vi "Project.vi"() -> ()   [LabVIEW 2014]
uses:
  Cntrls/Scada Mode.ctl
  Cntrls/Process Variable.ctl
  Cntrls/Manipulated Variable.ctl
  Cntrls/Message Cluster.ctl
  <vilib>/Utility/file.llb/Write To Spreadsheet File (DBL).vi
panel:
  in  "Начать запись":bool
  out "Waveform Graph 2":dbl[](graph)
  out "real-time, msec":dbl format="%#_4g"
  out "Initial graph and object identification graph":cluster{"all rows":dbl[], "all rows":dbl[]}[](graph) caption="Исходный\n график и\n график\n идентификации объекта"
  in  "dt, msec":u32=200
  in  "SCADA Start":bool
  in  "Exit Button":bool
  out "State":string caption="Display"
  in  "Tab Control":enum32{"SCADA", "Autotuning Controller"}(tab)
  in  "Pump MV":dbl(slide) scale=0.0..1.0
  in  "SCADA Configuration":T4={"HMI Selection"=enum."None", "Control Loop Mode"=enum."None", "Process Variable (PV)"=enum."Level", "Manipulated Variable (MV)"=enum."Pump"}
  out "PV, Level, [cm]":dbl
  in  "SP, Level Control, [cm]":dbl min=0.0 max=100.0 step=0.1
  in  "SP, Flow Control 2, [l/m]":dbl min=0.0 max=100.0 step=0.1
  out "PV, Flow meter 2, [l/m]":dbl format="%#_2g"
  in  "SP, Flow Control 1, [l/m]":dbl min=0.0 max=100.0 step=0.1
  in  "Valve 1 MV":dbl min=0.0 max=1.0 step=0.01
  out "Valve 1 Mode":enum16{"Auto", "Man", "Error"}(ring)
  out "Valve 2 Mode":enum16{"Auto", "Man", "Error"}(ring)
  in  "Working on closed valve 1 On/Off":bool
  out "LLA":bool
  in  "HHAS On/Off":bool
  out "HHA":bool
  in  "LLAS On/Off":bool
  in  "Valve 2 MV":dbl min=0.0 max=1.0 step=0.01
  out "OP, Valve 2%":dbl caption="%"
  out "?":string
  out "?":string
  out "Slide":dbl(slide) scale=0.0..30.0
  out "OP, Valve 1 %":dbl
  out "OP, Pump":dbl
  out "PV, Flow meter 1, [l/m]":dbl
  out "Pump Mode":enum16{"Auto", "Man", "Error"}(ring)
  out "Level N":dbl
  out "Flow meter N1":dbl
  out "Flow meterN2":dbl
  in  "Set PID Coeffs To PLC":bool
  in  "Start Identification":bool
  in  "Start Autotune":bool
  in  "Start Acquisition":bool
  in  "Control action level":dbl
  in  "Identified First - Order process + Deadtime transfer function":T5
  in  "P1":dbl
  in  "P2":dbl
  in  "P3":dbl
  in  "Transient response \nrecord ends in repetitions":dbl=50.0 min=50.0 max=300.0 step=1.0 format="%#_13g"
  in  "Select Identification Method":enum16{"Transient Response", "Proni"}(ring)
  in  "IMC filter value\n(PI > 0,7; PID > 1,7)":dbl(slide) step=0.1 scale=0.7..10.0
  in  "Select Autotune Method":enum32{"Ziegler  -  Nichols", "IMC", "Amigo"}(ring)
  in  "Type of controller":enum16{"PID", "PI", "P"}(ring)
  in  "Prony approximation zone":enum16{"3/4 zone", "1/2 zone", "1/3 zone"}(ring)
  out "Аverage error":dbl
  out "Transient response database":dbl[][](array[numeric])
  out "Identification X":dbl[](array[numeric])
  in  "Process Variable (PV)":T2
  in  "Manipulated Variable (MV)":T3
  out "Waveform Graph":dbl[](graph)
  # "Valve 2"
  # "Valve 2"
  # "Mode"
  # "[%]"
  # "Valve 1"
  # "MV"
  # "Mode"
  # "[%]"
  # "MV"
  # "PUMP"
  # "Mode"
  # "MV"
  # "Config Control Loop"
  # "Transient response database record & Transfer function identification configuration"
  # "Identification Configuration"
  # "Select variables"
  # "Record parameters"
  # "PID Autotune configuration & Controller parametrs"
  # "Controller parameters"
  # "Autotune selection"
  # "Created by ATM-21-01 (Dem, Shish, Destructor)"
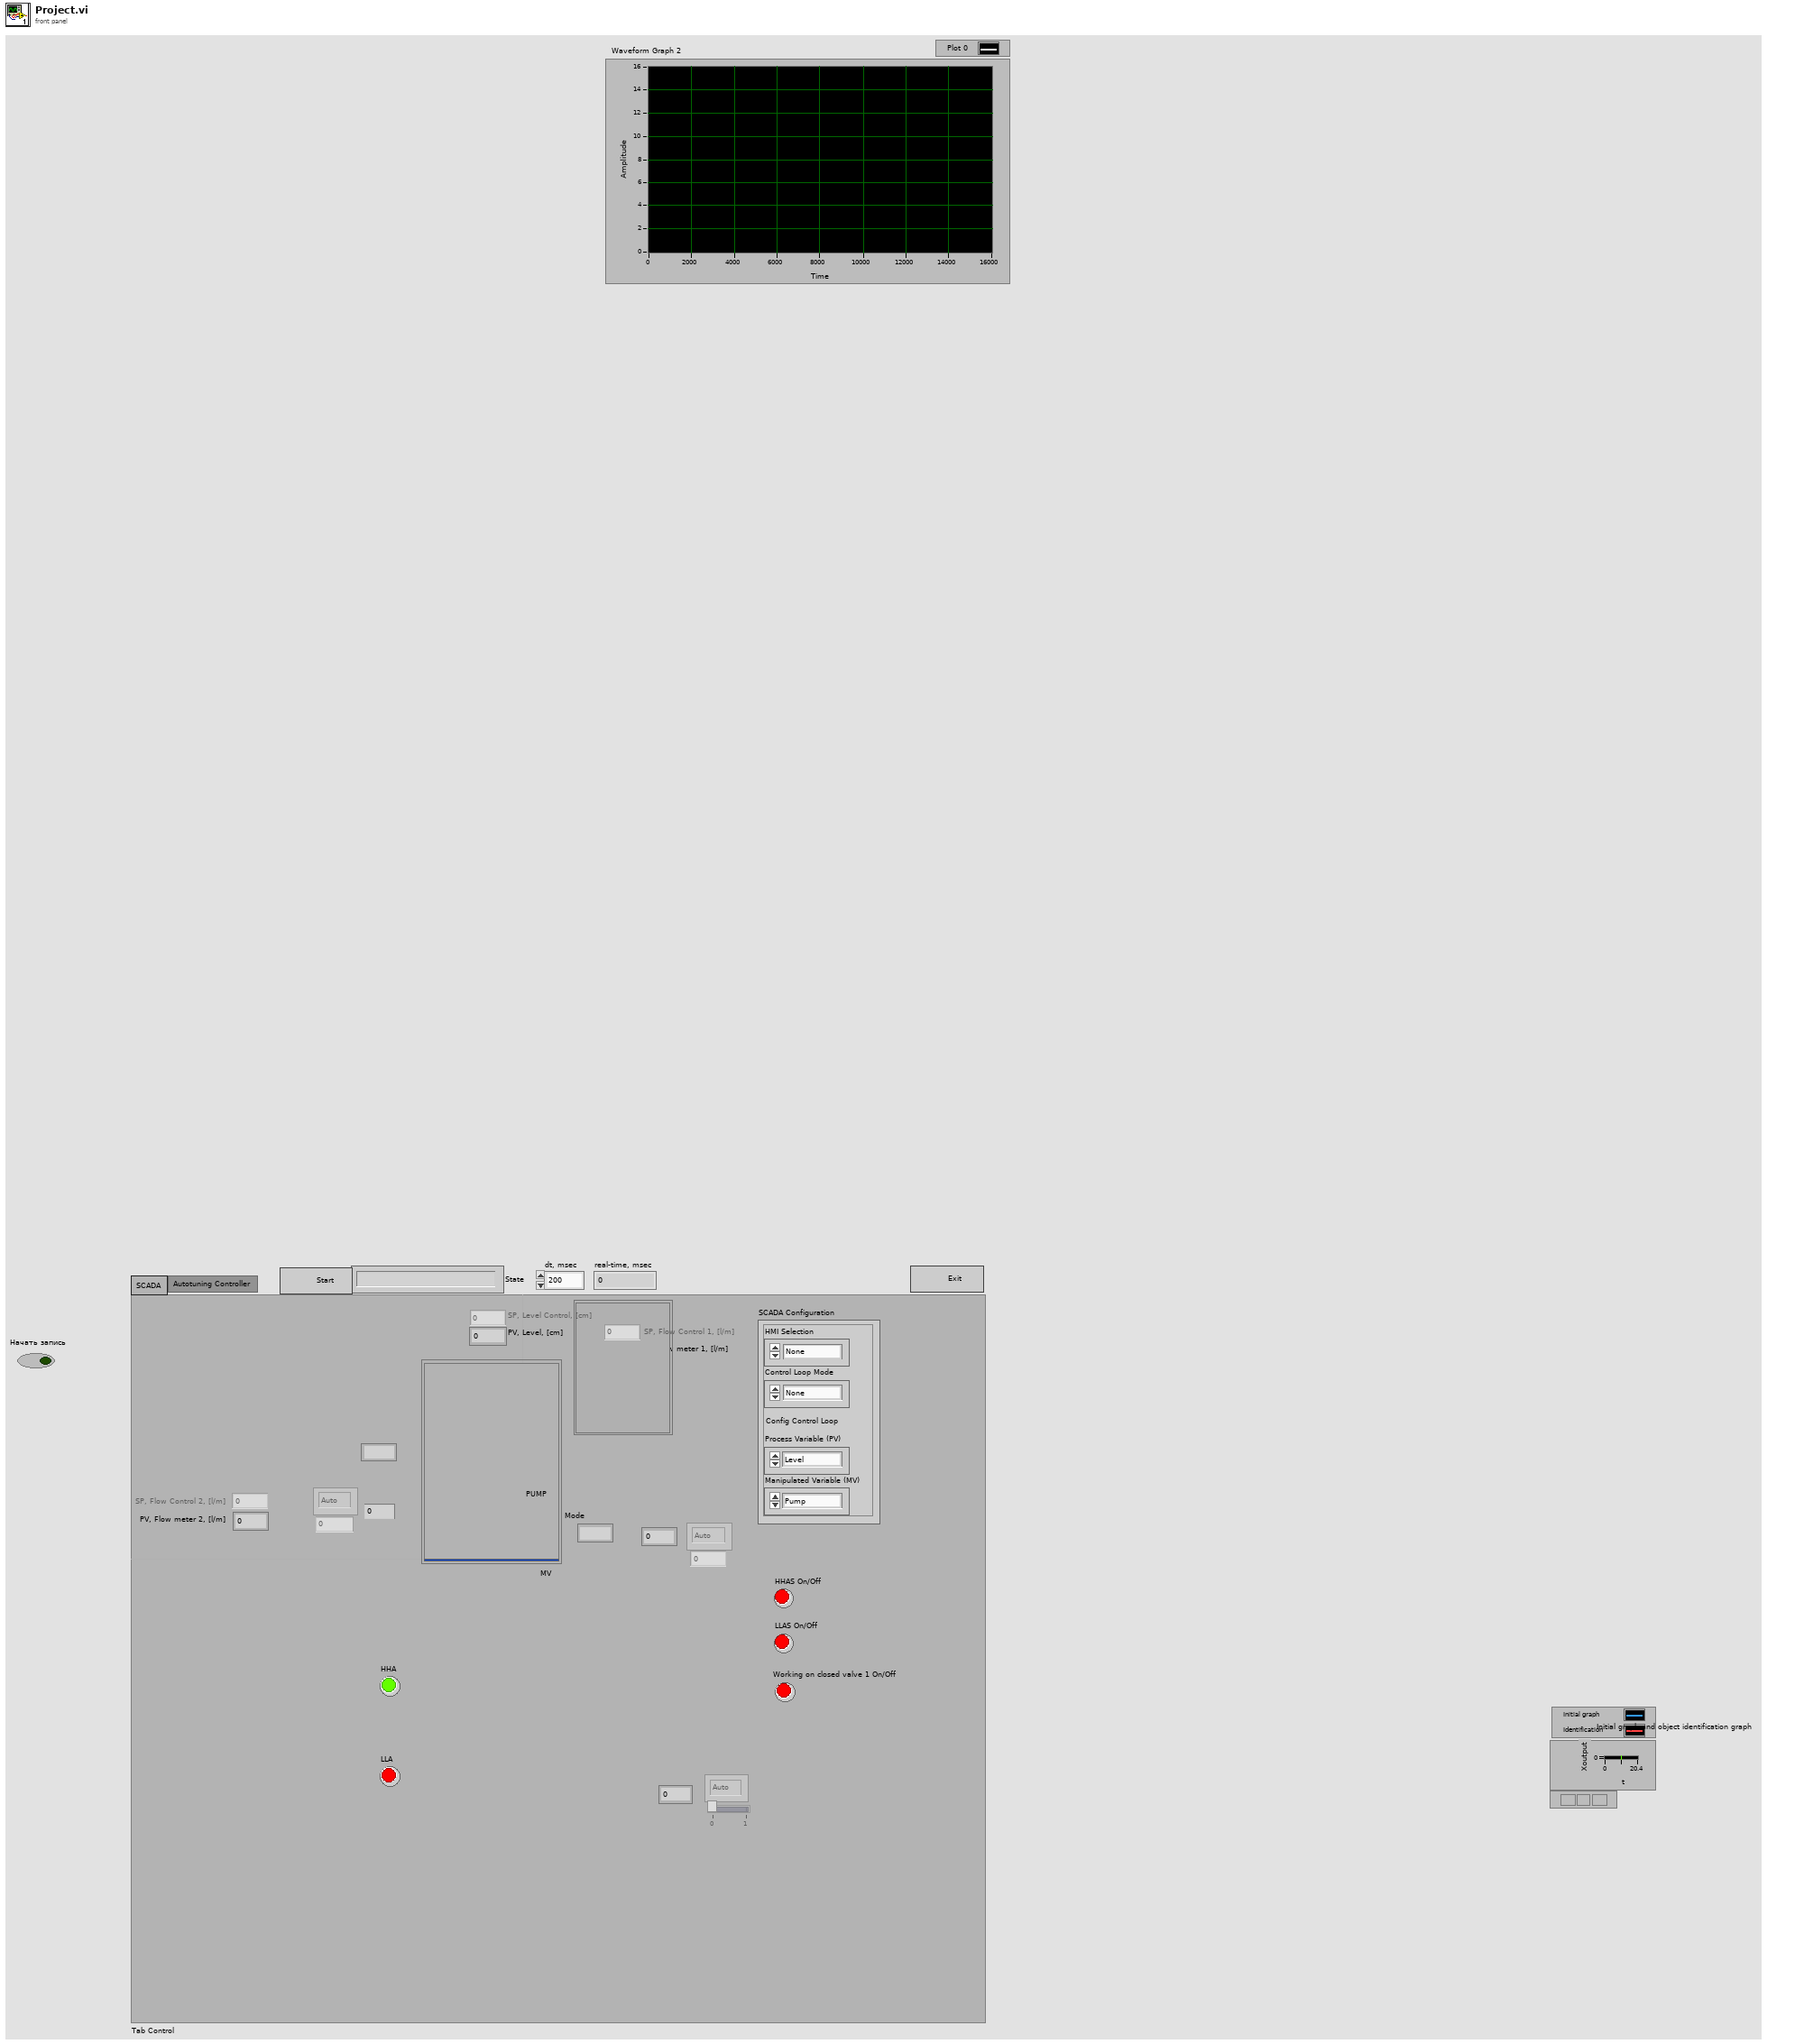
[diagram p1: front panel]
types:
  T1 = typedef "Scada Mode.ctl" = enum16{"None", "Manual", "Auto"}
  T2 = typedef "Process Variable.ctl" = enum16{"None", "Level", "Flow 1", "Flow 2"}
  T3 = typedef "Manipulated Variable.ctl" = enum16{"None", "Pump", "Valve 1", "Valve 2"}
  T4 = cluster{"HMI Selection":enum16{"Panel", "Scada", "Remote Control", "None"}, "Control Loop Mode":T1, "Process Variable (PV)":T2, "Manipulated Variable (MV)":T3}
  T5 = cluster{"K - gain coefficient":dbl, "tau - delay time":dbl, "T - time constant":dbl}
  T6 = typedef "Message Cluster.ctl" = cluster{"Enum":variant, "Message":string}
  T7 = enum16{"Read", "Write", "ReadWrite", "BufferedRead", "BufferedReadWrite"}
  T8 = cluster{"PVs":refnum<k13>[], "OPs":refnum<k13>[], "SPs":refnum<k13>[], "MVs":refnum<k13>[], "Controls":refnum<k13>[], "Indicators":refnum<k13>[], "Protection":refnum<k13>[], "PVs Norm ":refnum<k13>[]}
  T9 = enum16{"Panel", "Scada", "Remote Control", "None"}
  T10 = enum8{"Enabled", "Disabled", "Disabled and Grayed Out"}
  T11 = cluster{"к - gain coefficient":dbl, "tau -delay time":dbl, "T - time constant":dbl}
  T12 = cluster{"Data For Ident From OPC":dbl[], "Data For Ident From OPC":dbl[]}[]
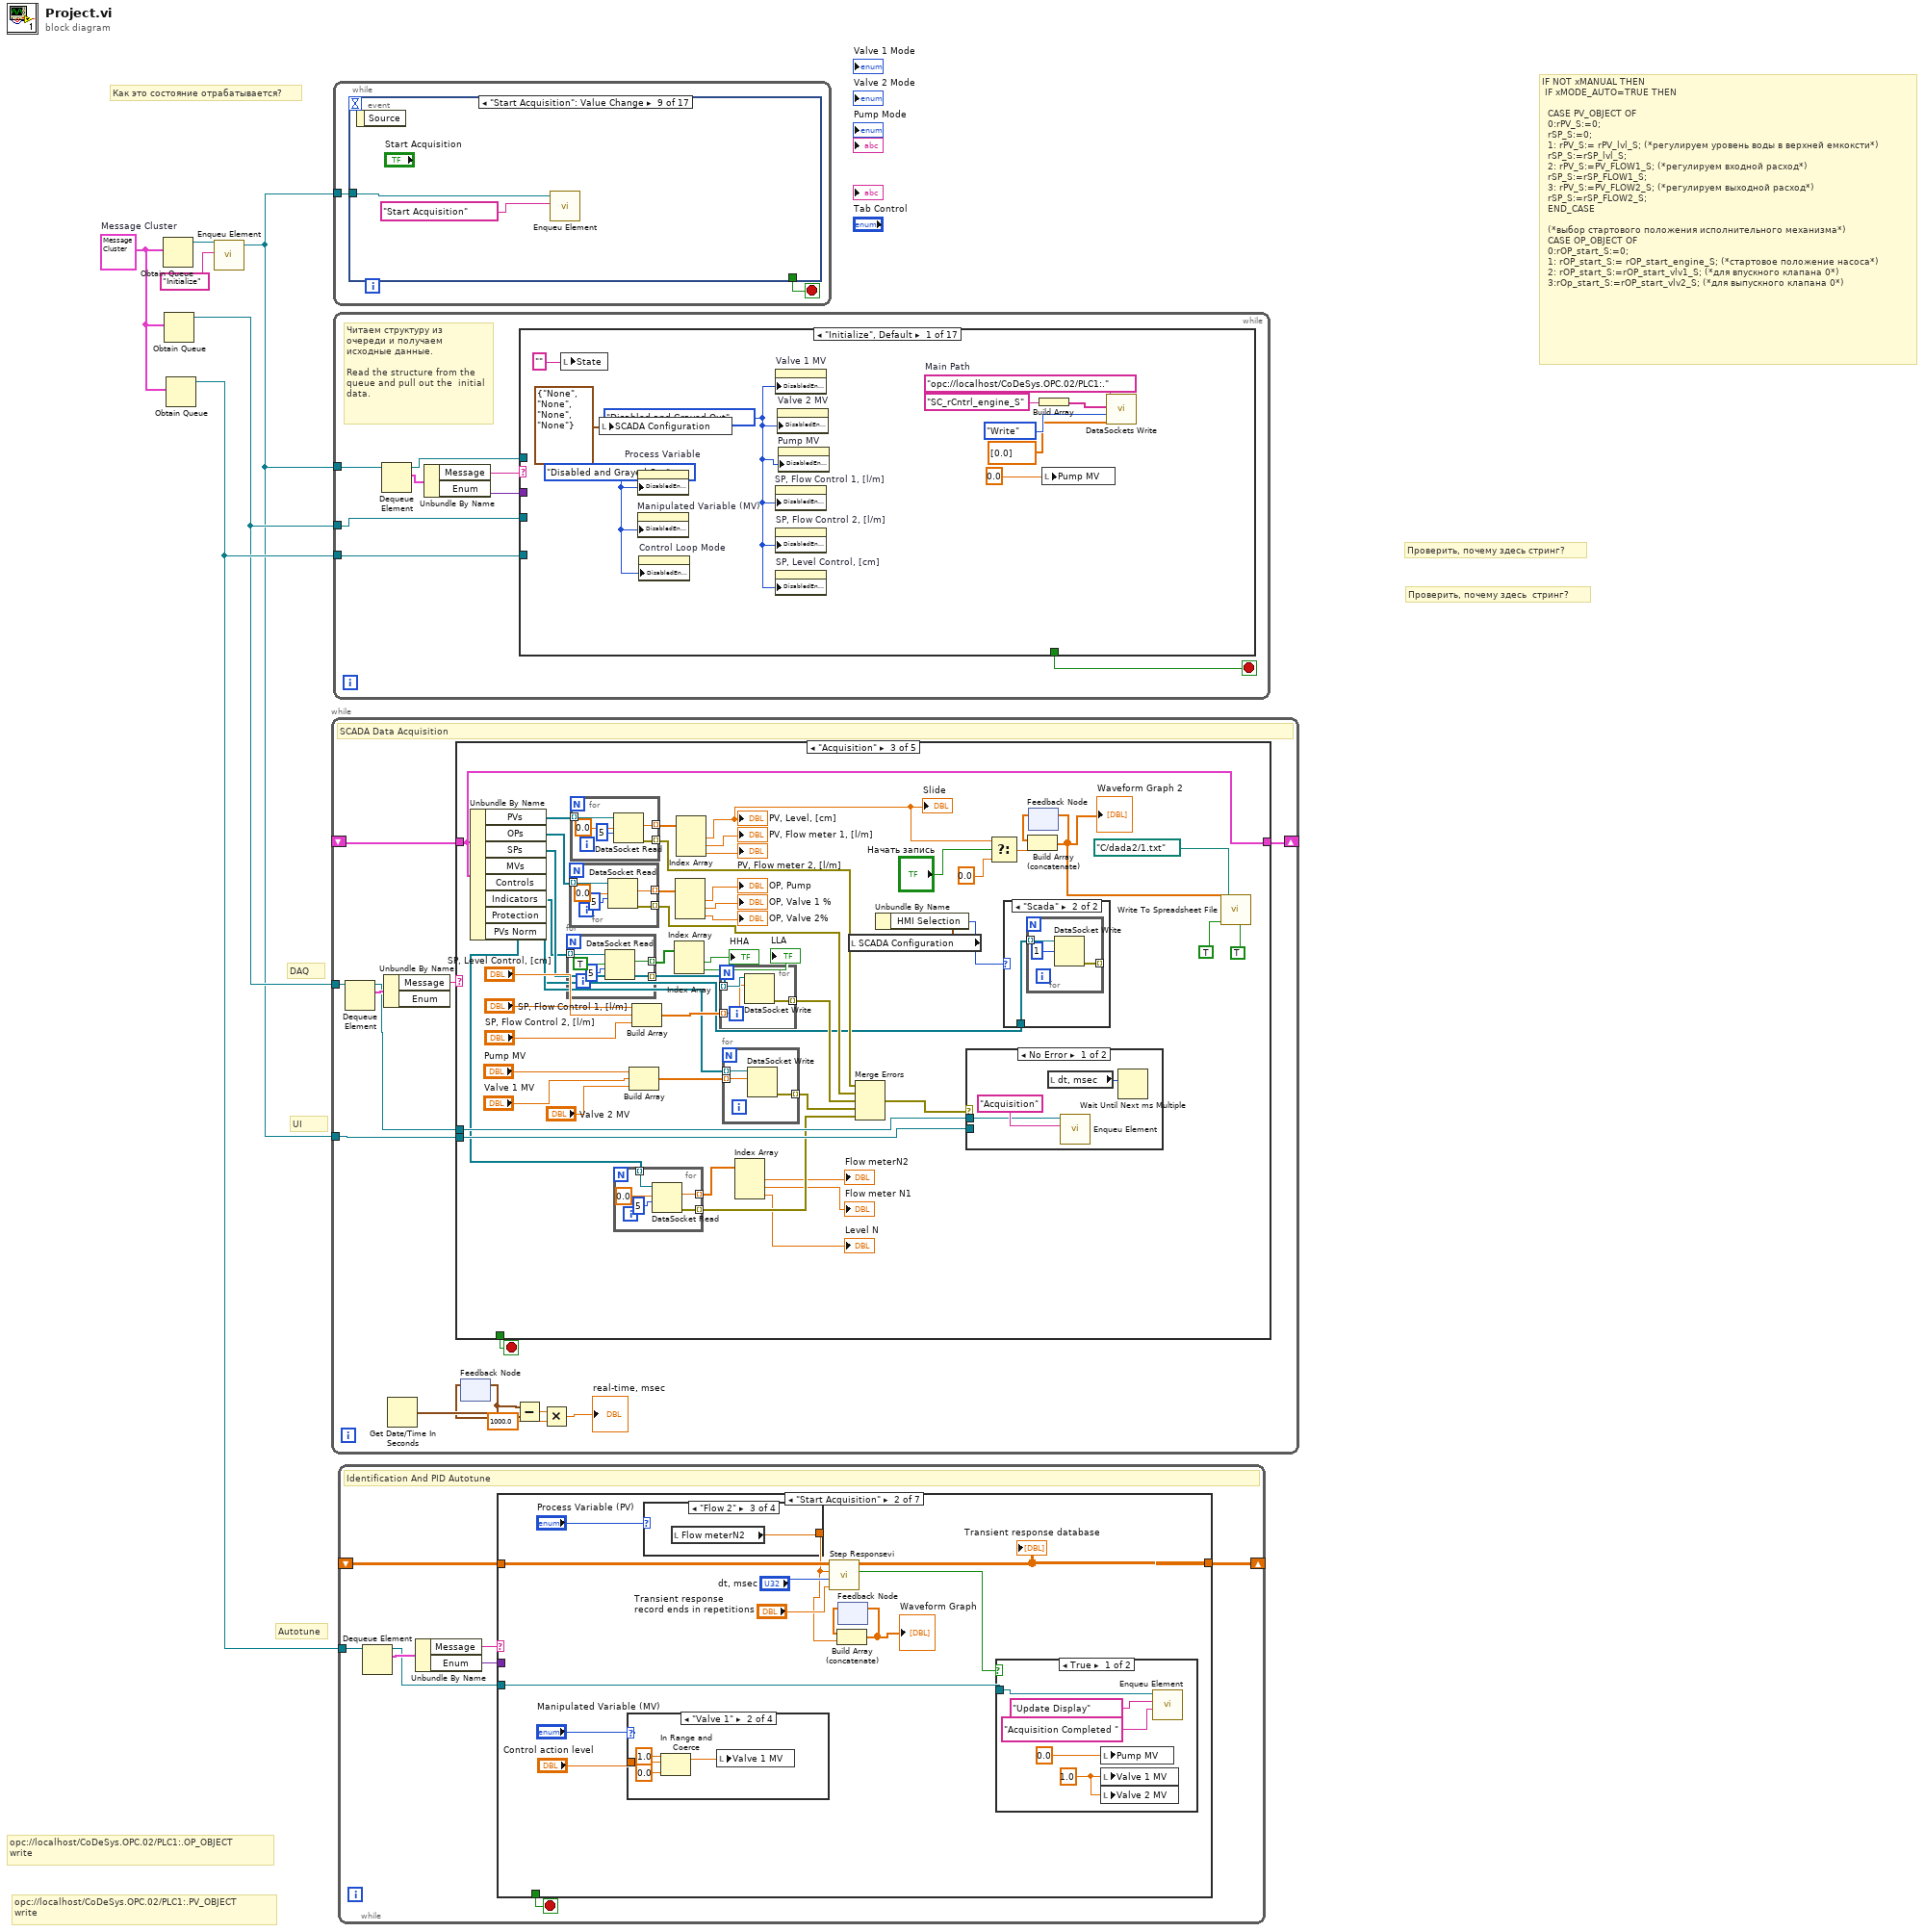
[diagram p0: block diagram]
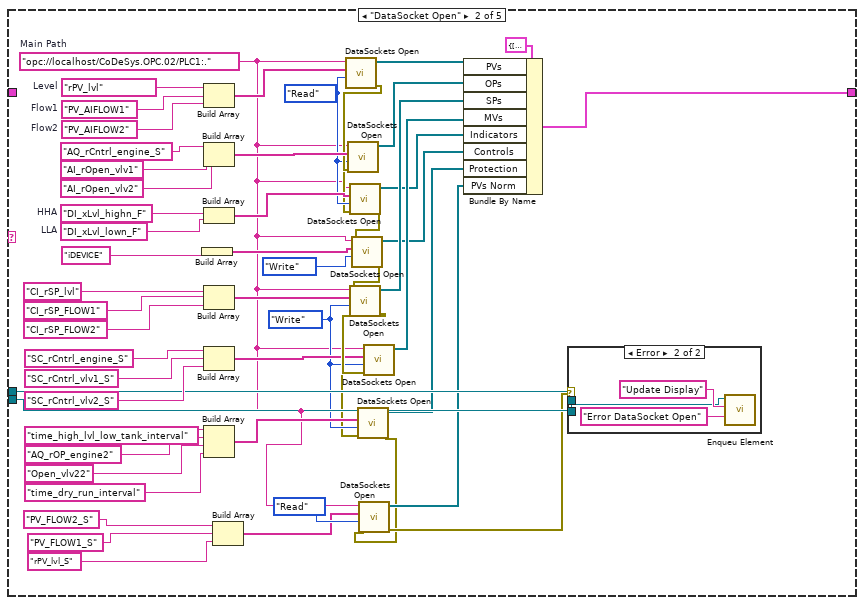
[diagram p3: hidden frame]
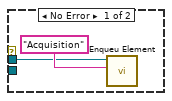
[diagram p4: hidden frame]
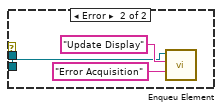
[diagram p6: hidden frame]
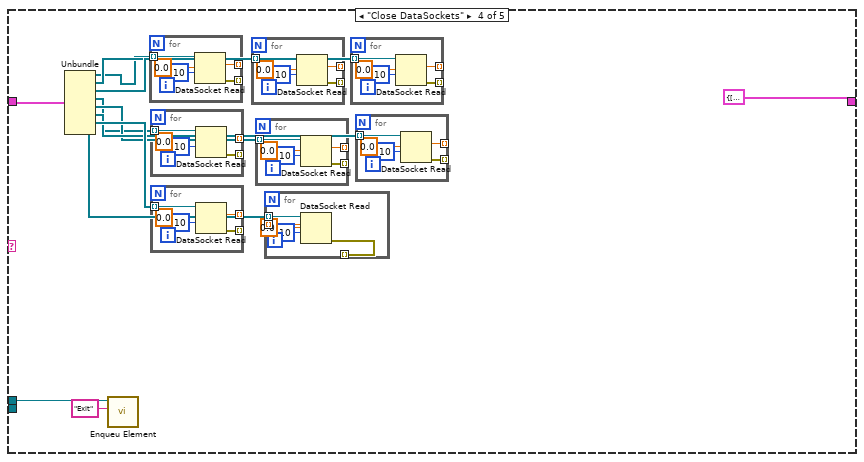
[diagram p7: hidden frame]
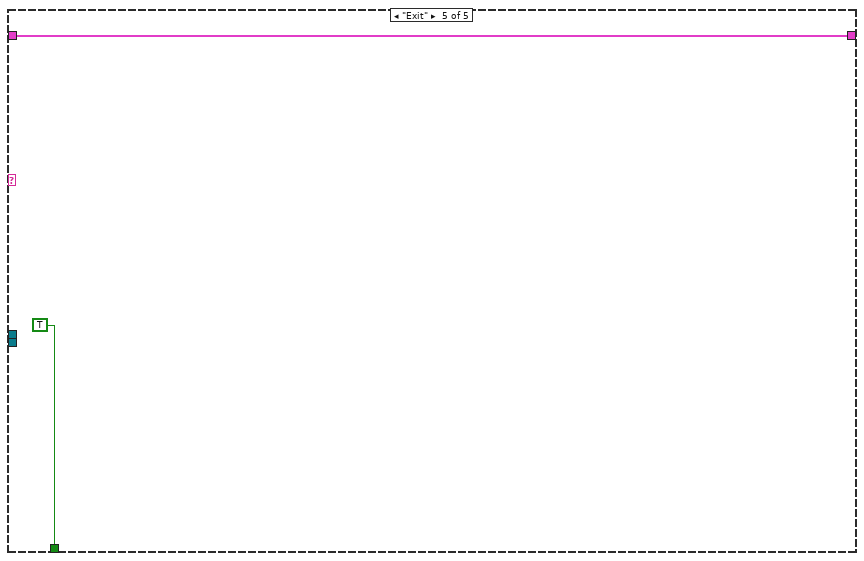
[diagram p8: hidden frame]
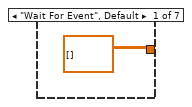
[diagram p9: hidden frame]
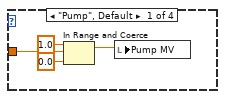
[diagram p10: hidden frame]
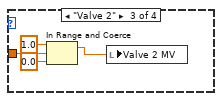
[diagram p11: hidden frame]
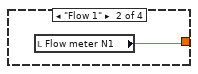
[diagram p14: hidden frame]
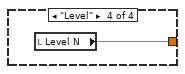
[diagram p15: hidden frame]
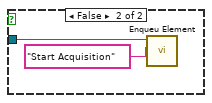
[diagram p16: hidden frame]
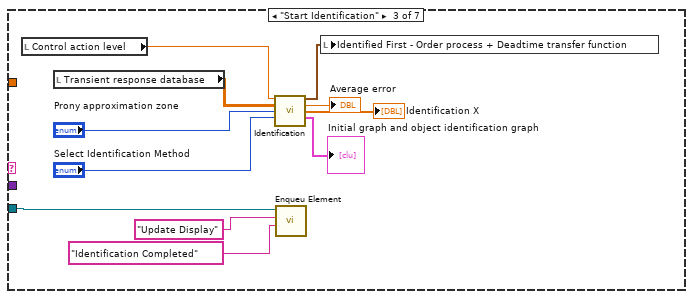
[diagram p17: hidden frame]
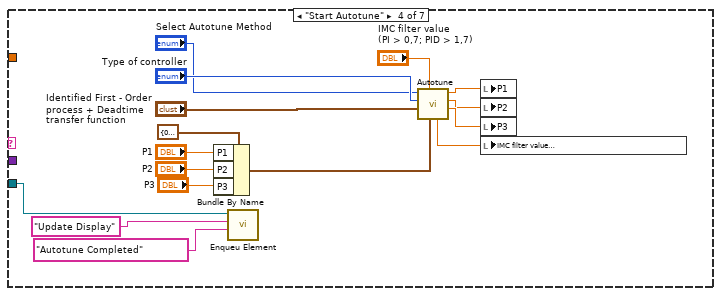
[diagram p18: hidden frame]
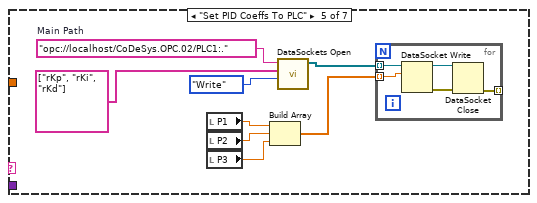
[diagram p19: hidden frame]
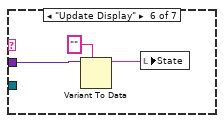
[diagram p20: hidden frame]
diagram:
  w3 = T6 {"Enum"=variant, "Message"=""}  # Message Cluster
  # "Проверить, почему здесь  стринг?"
  # "Проверить, почему здесь стринг?"
  # "IF NOT xMANUAL THEN\n\tIF xMODE_AUTO=TRUE THEN\n\n\t\tCASE PV_OBJECT OF\n\t\t0:rPV_S:=0;\n\t\trSP_S:=0;\n\t\t1: rPV_S:= rPV_lvl_S; (*регулируем уровень воды в верхней емкоксти*)\n\t\trSP_S:=rSP_lvl_S;\n\t\t2: rPV_S:=PV_FLOW1_S; (*регулируем входной расход*)\n\t\trSP_S:=rSP_FLOW1_S;\n\t\t3: rPV_S:=PV_FLOW2_S; (*регулируем выходной расход*)\n\t\trSP_S:=rSP_FLOW2_S;\n\t\tEND_CASE\n\n\t\t(*выбор стартового положения исполнительного механизма*)\n\t\tCASE OP_OBJECT OF\n\t\t0:rOP_start_S:=0;\n\t\t1: rOP_start_S:= rOP_start_engine_S; (*стартовое положение насоса*)\n\t\t2: rOP_start_S:=rOP_start_vlv1_S; (*для впускного клапана 0*)\n\t\t3:rOp_start_S:=rOP_start_vlv2_S; (*для выпускного клапана 0*)"
  # "Autotune"
  # "DAQ"
  # "UI"
  # "opc://localhost/CoDeSys.OPC.02/PLC1:.PV_OBJECT\nwrite"
  # "opc://localhost/CoDeSys.OPC.02/PLC1:.OP_OBJECT\nwrite"
  # "Как это состояние отрабатывается?"
  n1 = Obtain Queue(element data type=w3) -> (queue out=w5:refnum<queue>)  [unwired: 4 in, 2 out]
  n2 = Obtain Queue(element data type=w3) -> (queue out=w2:refnum<queue>)  [unwired: 4 in, 2 out]
  n3 = Obtain Queue(element data type=w3) -> (queue out=w6:refnum<queue>)  [unwired: 4 in, 2 out]
  n4 = call "Enqueu Element.vi"("Message"="Initialize", "Queue in"=w5) -> ("queue out"=w1:refnum<queue>)  [unwired: 9 in]
  n5 = while {
    tunnel: w2 -> [w17]
    shift-right: [w16] -> _
    shift-left: _ -> [w15]
    tunnel: w1 -> [w13]
    stop <- w14 stop-if-true
    # "SCADA Data Acquisition"
    n6 = Dequeue Element(queue=w17) -> (queue out=w12:refnum<queue>, element=w19:T6)  [unwired: 2 in, 2 out]
    n7 = Unbundle By Name(w19) -> ("Message"=w18:string)  [unwired: 1 out]
    n8 = Get Date/Time In Seconds() -> (seconds since 1Jan1904=w11:timestamp)
    n9 = case shown="\"Acquisition\"" w18 {
      tunnel: [w20 w66 w129 T8 {"PVs"=[], "OPs"=[], "SPs"=[], "MVs"=[], "Controls"=[], "Indicators"=[], "Protection"=[], "PVs Norm "=[]} ("cluster") w218] -> w16
      tunnel: w12 -> [_ w65 w105 w167 _]
      tunnel: w15 -> [w20 _ w129 w169 w218]
      tunnel: [_ _ _ _ TRUE] -> w14
      tunnel: w13 -> [_ w58 w104 _ _]
      frame "Wait For Event", Default {
      }
      frame "DataSocket Open" {
        w45 = "DI_xLvl_lown_F"  # LLA
        w46 = "DI_xLvl_highn_F"  # HHA
        w35 = T7."Write" ("mode")
        w42 = T7."Read" ("mode")
        w23 = "opc://localhost/CoDeSys.OPC.02/PLC1:."  # Main Path
        w56 = "PV_AIFLOW2"  # Flow2
        w57 = "PV_AIFLOW1"  # Flow1
        w75 = "rPV_lvl"  # Level
        n10 = Build Array("iDEVICE") -> (w51:string[])
        n11 = Build Array(w75, w57, w56) -> (w74:string[])
        n12 = Build Array("AQ_rCntrl_engine_S", "AI_rOpen_vlv1", "AI_rOpen_vlv2") -> (w63:string[])
        n13 = Build Array(w46, w45) -> (w43:string[])
        n14 = Build Array("CI_rSP_lvl", "CI_rSP_FLOW1", "CI_rSP_FLOW2") -> (w55:string[])
        n15 = Build Array("SC_rCntrl_engine_S", "SC_rCntrl_vlv1_S", "SC_rCntrl_vlv2_S") -> (w53:string[])
        n16 = Build Array("time_high_lvl_low_tank_interval", "AQ_rOP_engine2", "Open_vlv22", "time_dry_run_interval") -> (w36:string[])
        n17 = Build Array("PV_FLOW2_S", "PV_FLOW1_S", "rPV_lvl_S") -> (w24:string[])
        n18 = call "DataSockets Open.vi"("mode"=w42, "Variables"=w74, "Main Path"=w23) -> ("error out"=w62:errorcluster, "Array"=w64:refnum<k13>[])  [unwired: 7 in]
        n19 = call "DataSockets Open.vi"("error IO"=w62, "mode"=w42, "Variables"=w63, "Main Path"=w23) -> ("error out"=w41:errorcluster, "Array"=w61:refnum<k13>[])  [unwired: 6 in]
        n20 = call "DataSockets Open.vi"("error IO"=w41, "mode"=w42, "Variables"=w43, "Main Path"=w23) -> ("error out"=w31:errorcluster, "Array"=w40:refnum<k13>[])  [unwired: 6 in]
        n21 = call "DataSockets Open.vi"("error IO"=w31, "mode"=T7."Write", "Variables"=w51, "Main Path"=w23) -> ("error out"=w30:errorcluster, "Array"=w44:refnum<k13>[])  [unwired: 6 in]
        n22 = call "DataSockets Open.vi"("error IO"=w30, "mode"=w35, "Variables"=w55, "Main Path"=w23) -> ("error out"=w54:errorcluster, "Array"=w60:refnum<k13>[])  [unwired: 6 in]
        n23 = call "DataSockets Open.vi"("error IO"=w54, "mode"=w35, "Variables"=w53, "Main Path"=w23) -> ("error out"=w34:errorcluster, "Array"=w59:refnum<k13>[])  [unwired: 6 in]
        n24 = call "DataSockets Open.vi"("error IO"=w34, "mode"=w35, "Variables"=w36, "Main Path"=w23) -> ("error out"=w21:errorcluster, "Array"=w32:refnum<k13>[])  [unwired: 6 in]
        n25 = call "DataSockets Open.vi"("error IO"=w21, "mode"=T7."Read", "Variables"=w24, "Main Path"=w23) -> ("error out"=w26:errorcluster, "Array"=w22:refnum<k13>[])  [unwired: 6 in]
        n26 = Bundle By Name(cluster=T8 {"PVs"=[], "OPs"=[], "SPs"=[], "MVs"=[], "Controls"=[], "Indicators"=[], "Protection"=[], "PVs Norm "=[]}, "PVs"=w64, "OPs"=w61, "SPs"=w60, "MVs"=w59, "Indicators"=w40, "Controls"=w44, "Protection"=w32, "PVs Norm"=w22) -> (w66:T8)
        n27 = case shown="Error" w26 {
          tunnel: w65 -> [w76 _]
          tunnel: w58 -> [_ w78]
          frame No Error {
            n28 = call "Enqueu Element.vi"("Message"="Acquisition", "Queue in"=w76) -> ()  [unwired: 9 in, 1 out]
          }
          frame Error {
            n29 = call "Enqueu Element.vi"("Enum in"="Error DataSocket Open" ("Message"), "Message"="Update Display", "Queue in"=w78) -> ()  [unwired: 8 in, 1 out]
          }
        }
      }
      frame "Acquisition" {
        n30 = Unbundle By Name(w129) -> ("PVs"=w127:refnum<k13>[], "OPs"=w126:refnum<k13>[], "SPs"=w122:refnum<k13>[], "MVs"=w118:refnum<k13>[], "Controls"=w101:refnum<k13>[], "Indicators"=w100:refnum<k13>[], "PVs Norm"=w96:refnum<k13>[])  [unwired: 1 out]
        n31 = for {
          tunnel: w100 -> [w139] mode=indexing
          tunnel: [w138] -> w99 mode=indexing
          tunnel: [w136] -> _ mode=indexing
          n32 = DataSocket Read(9:5 ("ms timeout (10000)"), 10:TRUE, 11:w139) -> (0:w136:errorcluster, 2:w138:bool)  [unwired: 2 in, 5 out]
        }
        n33 = for {
          tunnel: w126 -> [w160] mode=indexing
          tunnel: [w159] -> w114 mode=indexing
          tunnel: [w156] -> w109 mode=indexing
          n34 = DataSocket Read(9:5 ("ms timeout (10000)"), 10:0.0, 11:w160) -> (0:w156:errorcluster, 2:w159:dbl)  [unwired: 2 in, 5 out]
        }
        n35 = for {
          tunnel: w127 -> [w165] mode=indexing
          tunnel: [w164] -> w117 mode=indexing
          tunnel: [w161] -> w110 mode=indexing
          n36 = DataSocket Read(9:5 ("ms timeout (10000)"), 10:0.0, 11:w165) -> (0:w161:errorcluster, 2:w164:dbl)  [unwired: 2 in, 5 out]
        }
        n37 = for {
          tunnel: [w134] -> w94 mode=indexing
          tunnel: [w132] -> w95 mode=indexing
          tunnel: w96 -> [w131] mode=indexing
          n38 = DataSocket Read(9:5 ("ms timeout (10000)"), 10:0.0, 11:w131) -> (0:w132:errorcluster, 2:w134:dbl)  [unwired: 2 in, 5 out]
        }
        n39 = Build Array("Pump MV", "Valve 1 MV", "Valve 2 MV") -> (w119:dbl[])
        n40 = Build Array("SP, Level Control, [cm]", "SP, Flow Control 1, [l/m]", "SP, Flow Control 2, [l/m]") -> (w121:dbl[])
        n41 = Index Array(array=w99) -> (element #1=→"HHA":bool, element #2=→"LLA":bool)  [unwired: 2 in]
        n42 = Index Array(array=w114) -> (element #1=→"OP, Pump":dbl, element #2=→"OP, Valve 1 %":dbl, element #3=→"OP, Valve 2%":dbl)  [unwired: 3 in]
        n43 = Index Array(array=w117) -> (element #1=w83:dbl, element #2=→"PV, Flow meter 1, [l/m]":dbl, element #3=→"PV, Flow meter 2, [l/m]":dbl)  [unwired: 3 in]
        "PV, Level, [cm]" <- w83
        "Slide" <- w83
        n44 = for {
          tunnel: w122 -> [w155] mode=indexing
          tunnel: w121 -> [w154] mode=indexing
          tunnel: [w153] -> w108 mode=indexing
          n45 = DataSocket Write(10:w154, 11:w155) -> (0:w153:errorcluster)  [unwired: 2 in, 2 out]
        }
        n46 = for {
          tunnel: w119 -> [w152] mode=indexing
          tunnel: w118 -> [w151] mode=indexing
          tunnel: [w150] -> w107 mode=indexing
          n47 = DataSocket Write(10:w152, 11:w151) -> (0:w150:errorcluster)  [unwired: 2 in, 2 out]
        }
        n48 = Index Array(array=w94) -> (element #1=→"Flow meterN2":dbl, element #2=→"Flow meter N1":dbl, element #3=→"Level N":dbl)  [unwired: 3 in]
        n49 = local read "SCADA Configuration"() -> (w103:T4)
        n50 = Merge Errors(w110, w109, w108, w107, w95) -> (w106:errorcluster)
        n51 = Unbundle By Name(w103) -> ("HMI Selection"=w102:T9)
        n52 = case shown="No Error" w106 {
          tunnel: w105 -> [w145 _]
          tunnel: w104 -> [_ w147]
          frame No Error {
            n53 = local read "dt, msec"() -> (w144:u32)
            n54 = call "Enqueu Element.vi"("Message"="Acquisition", "Queue in"=w145) -> ()  [unwired: 9 in, 1 out]
            n55 = Wait Until Next ms Multiple(millisecond multiple=w144) -> ()  [unwired: 1 out]
          }
          frame Error {
            n56 = call "Enqueu Element.vi"("Enum in"="Error Acquisition" ("Message"), "Message"="Update Display", "Queue in"=w147) -> ()  [unwired: 8 in, 1 out]
          }
        }
        n57 = Select(t=w83, s="Начать запись", f=0.0) -> (s? t:f=w84:dbl)
        n58 = case shown="\"Scada\"" w102 {
          tunnel: w101 -> [_ w140]
          frame "Panel", Default {
          }
          frame "Scada" {
            n59 = for {
              tunnel: w140 -> [w143] mode=indexing
              tunnel: [w142] -> _ mode=indexing
              n60 = DataSocket Write(10:1, 11:w143) -> (0:w142:errorcluster)  [unwired: 2 in, 2 out]
            }
          }
        }
        n61 = feedback #1() -> (w89:dbl[])  [unwired: 1 in]
        n62 = Build Array (concatenate)(w89, w84) -> (w87:dbl[])
        "Waveform Graph 2" <- w87
        n63 = feedback-in #1(w87) -> ()
        n64 = call-poly <vilib>:"Write To Spreadsheet File.vi"("transpose? (no:F)"=TRUE, "append to file? (new file:F)"=TRUE, "1D data"=w87, "file path (dialog if empty)"=path "C:/dada2/1.txt") -> ()  [unwired: 4 in, 1 out]
      }
      frame "Close DataSockets" {
        n65 = Unbundle(w169) -> ("PVs"=w170:refnum<k13>[], "OPs"=w171:refnum<k13>[], "SPs"=w172:refnum<k13>[], "MVs"=w173:refnum<k13>[], "Controls"=w174:refnum<k13>[], "Indicators"=w175:refnum<k13>[], "Protection"=w176:refnum<k13>[], "PVs Norm"=w177:refnum<k13>[])
        n66 = call "Enqueu Element.vi"("Message"="Exit", "Queue in"=w167) -> ()  [unwired: 9 in, 1 out]
        n67 = for {
          tunnel: w170 -> [w217] mode=indexing
          tunnel: [w216] -> _ mode=indexing
          tunnel: [w213] -> _ mode=indexing
          n68 = DataSocket Read(9:10 ("ms timeout (10000)"), 10:0.0, 11:w217) -> (0:w213:errorcluster, 2:w216:dbl)  [unwired: 2 in, 5 out]
        }
        n69 = for {
          tunnel: w173 -> [w202] mode=indexing
          tunnel: [w201] -> _ mode=indexing
          tunnel: [w198] -> _ mode=indexing
          n70 = DataSocket Read(9:10 ("ms timeout (10000)"), 10:0.0, 11:w202) -> (0:w198:errorcluster, 2:w201:dbl)  [unwired: 2 in, 5 out]
        }
        n71 = for {
          tunnel: w176 -> [w187] mode=indexing
          tunnel: [w186] -> _ mode=indexing
          tunnel: [w183] -> _ mode=indexing
          n72 = DataSocket Read(9:10 ("ms timeout (10000)"), 10:0.0, 11:w187) -> (0:w183:errorcluster, 2:w186:dbl)  [unwired: 2 in, 5 out]
        }
        n73 = for {
          tunnel: w171 -> [w212] mode=indexing
          tunnel: [w211] -> _ mode=indexing
          tunnel: [w208] -> _ mode=indexing
          n74 = DataSocket Read(9:10 ("ms timeout (10000)"), 10:0.0, 11:w212) -> (0:w208:errorcluster, 2:w211:dbl)  [unwired: 2 in, 5 out]
        }
        n75 = for {
          tunnel: w174 -> [w197] mode=indexing
          tunnel: [w196] -> _ mode=indexing
          tunnel: [w193] -> _ mode=indexing
          n76 = DataSocket Read(9:10 ("ms timeout (10000)"), 10:0.0, 11:w197) -> (0:w193:errorcluster, 2:w196:dbl)  [unwired: 2 in, 5 out]
        }
        n77 = for {
          tunnel: w177 -> [w182] mode=indexing
          tunnel: [w181] -> _ mode=indexing
          tunnel: [w178] -> _ mode=indexing
          n78 = DataSocket Read(9:10 ("ms timeout (10000)"), 10:0.0, 11:w182) -> (0:w178:errorcluster, 2:w181:dbl)  [unwired: 2 in, 5 out]
        }
        n79 = for {
          tunnel: w172 -> [w207] mode=indexing
          tunnel: [w206] -> _ mode=indexing
          tunnel: [w203] -> _ mode=indexing
          n80 = DataSocket Read(9:10 ("ms timeout (10000)"), 10:0.0, 11:w207) -> (0:w203:errorcluster, 2:w206:dbl)  [unwired: 2 in, 5 out]
        }
        n81 = for {
          tunnel: w175 -> [w192] mode=indexing
          tunnel: [w191] -> _ mode=indexing
          tunnel: [w188] -> _ mode=indexing
          n82 = DataSocket Read(9:10 ("ms timeout (10000)"), 10:0.0, 11:w192) -> (0:w188:errorcluster, 2:w191:dbl)  [unwired: 2 in, 5 out]
        }
      }
      frame "Exit" {
      }
    }
    n83 = feedback-in #2(w11) -> ()
    n84 = feedback #2() -> (w10:timestamp)  [unwired: 1 in]
    n85 = Subtract(x=w11, y=w10) -> (x-y=w9:dbl)
    n86 = Multiply(x=w9, y=1000.0) -> (x*y=→"real-time, msec":dbl)
  }
  n87 = while {
    tunnel: w1 -> [w220]
    stop <- w221 stop-if-true
    n88 = event shown="[8] \"Start Acquisition\": Value Change" {
      selector: _ -> [_ _ _ _ _ _ _ _ _ _ _ _ _ _ _ _ _]
      dyn-events: _ -> [_ _ _ _ _ _ _ _ _ _ _ _ _ _ _ _ _]
      timeout: _ -> [_ _ _ _ _ _ _ _ _ _ _ _ _ _ _ _ _]
      tunnel: [_ _ _ _ _ _ _ _ _ _ _ _ _ _ _ "Exit Button" _] -> w221
      tunnel: w220 -> [_ w225 w228 w230 w235 w239 w242 w244 w247 w248 w251 w254 w256 w259 w262 w264 _]
      event Timeout {
        n89 = event-data() -> ()  [unwired: 1 in, 1 out]
      }
      event "SCADA Configuration.HMI Selection": Value Change {
        n90 = event-data() -> ()  [unwired: 1 in, 1 out]
        n91 = local read "SCADA Configuration"() -> (w222:T4)
        n92 = Unbundle By Name(w222) -> ("HMI Selection"=w223:T9)
        n93 = call "Enqueu Element.vi"("Enum in"=w223, "Message"="HMI Selection", "Queue in"=w225) -> ()  [unwired: 8 in, 1 out]
      }
      event Value Change {
        n94 = event-data() -> ()  [unwired: 1 in, 1 out]
        n95 = Unbundle By Name("SCADA Configuration") -> ("Control Loop Mode"=w226:T1)
        n96 = call "Enqueu Element.vi"("Enum in"=w226, "Message"="Control Loop Mode", "Queue in"=w228) -> ()  [unwired: 8 in, 1 out]
      }
      event "SCADA Start": Value Change {
        n97 = event-data() -> ()  [unwired: 1 in, 2 out]
        n98 = call "Enqueu Element.vi"("Message"="SCADA Start", "Queue in"=w230) -> ()  [unwired: 9 in, 1 out]
      }
      event Value Change {
        n99 = event-data() -> ()  [unwired: 1 in, 1 out]
        n100 = local read "SCADA Configuration"() -> (w233:T4)
        n101 = Unbundle By Name(w233) -> ("Process Variable (PV)"=w232:T2)
        n102 = call "Enqueu Element.vi"("Enum in"=w232, "Message"="PV Select", "Queue in"=w235) -> ()  [unwired: 8 in, 1 out]
      }
      event Value Change {
        n103 = event-data() -> ()  [unwired: 1 in, 1 out]
        n104 = local read "SCADA Configuration"() -> (w237:T4)
        n105 = Unbundle By Name(w237) -> ("Manipulated Variable (MV)"=w236:T3)
        n106 = call "Enqueu Element.vi"("Enum in"=w236, "Message"="MV Select", "Queue in"=w239) -> ()  [unwired: 8 in, 1 out]
      }
      event "LLAS On/Off": Value Change {
        n107 = event-data() -> ()  [unwired: 1 in, 1 out]
        n108 = call "Enqueu Element.vi"("Enum in"="LLAS On/Off", "Message"="Down", "Queue in"=w242) -> ()  [unwired: 8 in, 1 out]
      }
      event "Working on closed valve 1 On/Off": Value Change {
        n109 = event-data() -> ()  [unwired: 1 in, 6 out]
        n110 = call "Enqueu Element.vi"("Enum in"="Working on closed valve 1 On/Off", "Message"="PumpDefence", "Queue in"=w244) -> ()  [unwired: 8 in, 1 out]
      }
      event "Start Acquisition": Value Change {
        n111 = event-data() -> ()  [unwired: 1 in, 1 out]
        n112 = call "Enqueu Element.vi"("Message"="Start Acquisition", "Queue in"=w247) -> ()  [unwired: 9 in, 1 out]
      }
      event "Start Identification": Value Change {
        n113 = event-data() -> ()  [unwired: 1 in, 1 out]
        n114 = call "Enqueu Element.vi"("Message"="Start Identification", "Queue in"=w248) -> ()  [unwired: 9 in, 1 out]
      }
      event "Start Autotune": Value Change {
        n115 = event-data() -> ()  [unwired: 1 in, 1 out]
        n116 = call "Enqueu Element.vi"("Message"="Start Autotune", "Queue in"=w251) -> ()  [unwired: 9 in, 1 out]
      }
      event "HHAS On/Off": Value Change {
        n117 = event-data() -> ()  [unwired: 1 in, 1 out]
        n118 = call "Enqueu Element.vi"("Enum in"="HHAS On/Off", "Message"="Up", "Queue in"=w254) -> ()  [unwired: 8 in, 1 out]
      }
      event "Select Identification Method": Value Change {
        n119 = event-data() -> ()  [unwired: 1 in, 1 out]
        n120 = local read "Select Identification Method"() -> (w255:enum16{"Transient Response", "Proni"})
        n121 = call "Enqueu Element.vi"("Enum in"=w255, "Message"="Id method", "Queue in"=w256) -> ()  [unwired: 8 in, 1 out]
      }
      event "Select Autotune Method": Value Change {
        n122 = event-data() -> ()  [unwired: 1 in, 3 out]
        n123 = local read "Select Autotune Method"() -> (w258:enum32{"Ziegler  -  Nichols", "IMC", "Amigo"})
        n124 = call "Enqueu Element.vi"("Enum in"=w258, "Message"="Auto method", "Queue in"=w259) -> ()  [unwired: 8 in, 1 out]
      }
      event "Set PID Coeffs To PLC": Value Change {
        n125 = event-data() -> ()  [unwired: 1 in, 2 out]
        n126 = call "Enqueu Element.vi"("Message"="Set PID Coeffs To PLC", "Queue in"=w262) -> ()  [unwired: 9 in, 1 out]
      }
      event "Exit Button": Value Change {
        n127 = event-data() -> ()  [unwired: 1 in, 1 out]
        n128 = call "Enqueu Element.vi"("Message"="Exit", "Queue in"=w264) -> ()  [unwired: 9 in, 1 out]
      }
      event Panel Close? {
        n129 = event-data() -> ()  [unwired: 1 in, 4 out]
        n130 = event-data() -> ()  [unwired: 2 in, 1 out]
      }
    }
  }
  n131 = while {
    tunnel: w1 -> [w272]
    tunnel: w6 -> [w268]
    tunnel: w2 -> [w266]
    stop <- w273 stop-if-true
    # "Читаем структуру из \nочереди и получаем\nисходные данные.\n\nRead the structure from the queue and pull out the  initial data."
    n132 = Dequeue Element(queue=w272) -> (queue out=w267:refnum<queue>, element=w271:T6)  [unwired: 2 in, 2 out]
    n133 = Unbundle By Name(w271) -> ("Message"=w270:string, "Enum"=w269:variant)
    n134 = case shown="\"Initialize\", Default" w270 {
      selector: w270 -> [_ _ _ _ _ w371 _ _ _ w412 w416 w420 w425 _ _ _ w444]
      tunnel: [_ _ _ _ _ _ _ _ _ _ _ _ _ _ _ _ w443] -> w273
      tunnel: w269 -> [_ w292 w299 w320 w340 _ w375 w388 w401 _ _ _ _ w430 w432 w437 _]
      tunnel: w268 -> [_ _ _ _ _ _ _ _ _ w415 w417 w421 w424 _ _ _ w445]
      tunnel: w267 -> [_ _ _ _ _ w372 _ _ _ w414 w418 w422 w426 _ _ _ _]
      tunnel: w266 -> [_ _ _ _ _ w374 _ _ _ _ _ _ _ _ _ _ w446]
      frame "Initialize", Default {
        w277 = "opc://localhost/CoDeSys.OPC.02/PLC1:."  # Main Path
        w274 = T10."Disabled and Grayed Out" ("Disabled")
        w281 = T10."Disabled and Grayed Out" ("Disabled")
        n135 = local write "State"("" ("Display")) -> ()
        n136 = local write "SCADA Configuration"(T4 {"HMI Selection"=enum."None", "Control Loop Mode"=enum."None", "Process Variable (PV)"=enum."None", "Manipulated Variable (MV)"=enum."None"} ("SCADA Controls")) -> ()
        n137 = property on="Process Variable" class="Enum (strict)"("DisabledEnum"=w281) -> ()  [unwired: 2 in, 2 out]
        n138 = property on="Manipulated Variable (MV)" class="Enum (strict)"("DisabledEnum"=w281) -> ()  [unwired: 2 in, 2 out]
        n139 = property on="Control Loop Mode" class="Enum (strict)"("DisabledEnum"=w281) -> ()  [unwired: 2 in, 2 out]
        n140 = property on="Valve 1 MV" class="DigNum (strict)"("DisabledEnum"=w274) -> ()  [unwired: 2 in, 2 out]
        n141 = property on="SP, Flow Control 1, [l/m]" class="DigNum (strict)"("DisabledEnum"=w274) -> ()  [unwired: 2 in, 2 out]
        n142 = property on="SP, Flow Control 2, [l/m]" class="DigNum (strict)"("DisabledEnum"=w274) -> ()  [unwired: 2 in, 2 out]
        n143 = property on="SP, Level Control, [cm]" class="DigNum (strict)"("DisabledEnum"=w274) -> ()  [unwired: 2 in, 2 out]
        n144 = property on="Valve 2 MV" class="DigNum (strict)"("DisabledEnum"=w274) -> ()  [unwired: 2 in, 2 out]
        n145 = property on="Pump MV" class="Slide (strict)"("DisabledEnum"=w274) -> ()  [unwired: 2 in, 2 out]
        n146 = Build Array("SC_rCntrl_engine_S") -> (w280:string[])
        n147 = local write "Pump MV"(0.0 ("Pump MV")) -> ()
        n148 = call "DataSockets Write.vi"("Data"=dbl[] [0.0], "mode"=T7."Write", "Array"=w280, "Main Path"=w277) -> ()  [unwired: 7 in, 1 out]
      }
      frame "HMI Selection" {
        w290 = "opc://localhost/CoDeSys.OPC.02/PLC1:."  # Main Path
        n149 = Variant To Data(type=0, Variant=w292) -> (data=w286:i32)  [unwired: 1 in, 1 out]
        n150 = Build Array(w286) -> (w285:i32[])
        n151 = Build Array("iDEVICE" ("PV")) -> (w289:string[])
        n152 = call "DataSockets Write.vi"("Data"=w285, "mode"=T7."Write", "Array"=w289, "Main Path"=w290) -> ()  [unwired: 7 in, 1 out]
        n153 = property on="Control Loop Mode" class="Enum (strict)"("DisabledEnum"=T10."Enabled" ("Disabled")) -> ()  [unwired: 2 in, 2 out]
      }
      frame "Control Loop Mode" {
        w296 = "opc://localhost/CoDeSys.OPC.02/PLC1:."  # Main Path
        n154 = Variant To Data(type=Scada_Mode."None" ("SCADA Mode"), Variant=w299) -> (data=w300:T1)  [unwired: 1 in, 1 out]
        n155 = case shown="\"Auto\"" w300 {
          tunnel: [bool[] [FALSE] bool[] [TRUE] bool[] [FALSE]] -> w293
          frame "Manual" {
            w303 = T10."Disabled and Grayed Out" ("Disabled")
            w301 = T10."Enabled" ("Disabled")
            w305 = enum16{"Auto", "Man", "Error"}."Man" ("Valve 1 Mode")
            w304 = T10."Disabled and Grayed Out" ("Disabled")
            n156 = property on="Valve 1 Mode" class="Enum (strict)"("Value"=w305) -> ()  [unwired: 2 in, 2 out]
            n157 = property on="Valve 2 Mode" class="Enum (strict)"("Value"=w305) -> ()  [unwired: 2 in, 2 out]
            n158 = property on="Pump Mode" class="Enum (strict)"("Value"=w305) -> ()  [unwired: 2 in, 2 out]
            n159 = property on="Valve 1 Mode" class="Enum (strict)"("DisabledEnum"=w304) -> ()  [unwired: 2 in, 2 out]
            n160 = property on="Valve 2 Mode" class="Enum (strict)"("DisabledEnum"=w304) -> ()  [unwired: 2 in, 2 out]
            n161 = property on="Pump Mode" class="Enum (strict)"("DisabledEnum"=w304) -> ()  [unwired: 2 in, 2 out]
            n162 = property on="Valve 1 MV" class="DigNum (strict)"("DisabledEnum"=w301) -> ()  [unwired: 2 in, 2 out]
            n163 = property on="SP, Flow Control 1, [l/m]" class="DigNum (strict)"("DisabledEnum"=w301) -> ()  [unwired: 2 in, 2 out]
            n164 = property on="SP, Flow Control 2, [l/m]" class="DigNum (strict)"("DisabledEnum"=w301) -> ()  [unwired: 2 in, 2 out]
            n165 = property on="SP, Level Control, [cm]" class="DigNum (strict)"("DisabledEnum"=w301) -> ()  [unwired: 2 in, 2 out]
            n166 = property on="Pump MV" class="Slide (strict)"("DisabledEnum"=w301) -> ()  [unwired: 2 in, 2 out]
            n167 = property on="Valve 2 MV" class="DigNum (strict)"("DisabledEnum"=w301) -> ()  [unwired: 2 in, 2 out]
            n168 = property on="Manipulated Variable (MV)" class="Enum (strict)"("DisabledEnum"=w303) -> ()  [unwired: 2 in, 2 out]
            n169 = property on="Process Variable" class="Enum (strict)"("DisabledEnum"=w303) -> ()  [unwired: 2 in, 2 out]
            n170 = property on="SP, Flow Control 1, [l/m]" class="DigNum (strict)"("DisabledEnum"=w303) -> ()  [unwired: 2 in, 2 out]
            n171 = property on="SP, Flow Control 2, [l/m]" class="DigNum (strict)"("DisabledEnum"=w303) -> ()  [unwired: 2 in, 2 out]
            n172 = property on="SP, Level Control, [cm]" class="DigNum (strict)"("DisabledEnum"=w303) -> ()  [unwired: 2 in, 2 out]
          }
          frame "Auto" {
            w306 = T10."Disabled and Grayed Out" ("Disabled")
            w308 = T10."Enabled" ("Disabled")
            n173 = property on="Process Variable" class="Enum (strict)"("DisabledEnum"=w308) -> ()  [unwired: 2 in, 2 out]
            n174 = property on="Manipulated Variable (MV)" class="Enum (strict)"("DisabledEnum"=w308) -> ()  [unwired: 2 in, 2 out]
            n175 = property on="Process Variable" class="Enum (strict)"("Value"=Process_Variable."None" ("Process Variable")) -> ()  [unwired: 2 in, 2 out]
            n176 = property on="Manipulated Variable (MV)" class="Enum (strict)"("Value"=Manipulated_Variable."None" ("Manipulated Variable (MV)")) -> ()  [unwired: 2 in, 2 out]
            n177 = property on="Valve 1 MV" class="DigNum (strict)"("DisabledEnum"=w306) -> ()  [unwired: 2 in, 2 out]
            n178 = property on="SP, Flow Control 1, [l/m]" class="DigNum (strict)"("DisabledEnum"=w306) -> ()  [unwired: 2 in, 2 out]
            n179 = property on="SP, Flow Control 2, [l/m]" class="DigNum (strict)"("DisabledEnum"=w306) -> ()  [unwired: 2 in, 2 out]
            n180 = property on="SP, Level Control, [cm]" class="DigNum (strict)"("DisabledEnum"=w306) -> ()  [unwired: 2 in, 2 out]
            n181 = property on="Valve 2 MV" class="DigNum (strict)"("DisabledEnum"=w306) -> ()  [unwired: 2 in, 2 out]
            n182 = property on="Pump MV" class="Slide (strict)"("DisabledEnum"=w306) -> ()  [unwired: 2 in, 2 out]
          }
          frame "None", Default {
            w312 = T10."Disabled and Grayed Out" ("Disabled")
            n183 = property on="SP, Flow Control 1, [l/m]" class="DigNum (strict)"("DisabledEnum"=w312) -> ()  [unwired: 2 in, 2 out]
            n184 = property on="SP, Flow Control 2, [l/m]" class="DigNum (strict)"("DisabledEnum"=w312) -> ()  [unwired: 2 in, 2 out]
            n185 = property on="SP, Level Control, [cm]" class="DigNum (strict)"("DisabledEnum"=w312) -> ()  [unwired: 2 in, 2 out]
          }
        }
        n186 = Build Array("xMODE_AUTO" ("PV")) -> (w295:string[])
        n187 = call "DataSockets Write.vi"("Data"=w293, "mode"=T7."Write", "Array"=w295, "Main Path"=w296) -> ()  [unwired: 7 in, 1 out]
      }
      frame "PV Select" {
        w316 = "opc://localhost/CoDeSys.OPC.02/PLC1:."  # Main Path
        n188 = Variant To Data(type=Process_Variable."None" ("Process Variable"), Variant=w320) -> (data=w319:T2)  [unwired: 1 in, 1 out]
        n189 = case shown="\"Flow 1\"" w319 {
          tunnel: [string[] ["0"] string[] ["2"] string[] ["3"] string[] ["1"]] -> w313
          frame "None", Default {
          }
          frame "Flow 1" {
            w323 = T10."Disabled and Grayed Out" ("Disabled")
            n190 = property on="SP, Flow Control 1, [l/m]" class="DigNum (strict)"("DisabledEnum"=T10."Enabled" ("Disabled")) -> ()  [unwired: 2 in, 2 out]
            n191 = property on="SP, Flow Control 2, [l/m]" class="DigNum (strict)"("DisabledEnum"=w323) -> ()  [unwired: 2 in, 2 out]
            n192 = property on="SP, Level Control, [cm]" class="DigNum (strict)"("DisabledEnum"=w323) -> ()  [unwired: 2 in, 2 out]
          }
          frame "Flow 2" {
            n193 = property on="SP, Flow Control 1, [l/m]" class="DigNum (strict)"("DisabledEnum"=T10."Disabled and Grayed Out" ("Disabled")) -> ()  [unwired: 2 in, 2 out]
            n194 = property on="SP, Flow Control 2, [l/m]" class="DigNum (strict)"("DisabledEnum"=T10."Enabled" ("Disabled")) -> ()  [unwired: 2 in, 2 out]
            n195 = property on="SP, Level Control, [cm]" class="DigNum (strict)"("DisabledEnum"=T10."Disabled and Grayed Out" ("Disabled")) -> ()  [unwired: 2 in, 2 out]
          }
          frame "Level" {
            n196 = property on="SP, Flow Control 1, [l/m]" class="DigNum (strict)"("DisabledEnum"=T10."Disabled and Grayed Out" ("Disabled")) -> ()  [unwired: 2 in, 2 out]
            n197 = property on="SP, Flow Control 2, [l/m]" class="DigNum (strict)"("DisabledEnum"=T10."Disabled and Grayed Out" ("Disabled")) -> ()  [unwired: 2 in, 2 out]
            n198 = property on="SP, Level Control, [cm]" class="DigNum (strict)"("DisabledEnum"=T10."Enabled" ("Disabled")) -> ()  [unwired: 2 in, 2 out]
          }
        }
        n199 = Build Array("PV_OBJECT" ("PV")) -> (w315:string[])
        n200 = call "DataSockets Write.vi"("Data"=w313, "mode"=T7."Write", "Array"=w315, "Main Path"=w316) -> ()  [unwired: 7 in, 1 out]
      }
      frame "MV Select" {
        w337 = "opc://localhost/CoDeSys.OPC.02/PLC1:."  # Main Path
        n201 = Variant To Data(type=Manipulated_Variable."None" ("Manipulated Variable (MV)"), Variant=w340) -> (data=w339:T3)  [unwired: 1 in, 1 out]
        n202 = case shown="\"None\", Default" w339 {
          tunnel: [string[] ["1"] string[] ["2"] string[] ["3"] string[] ["0"]] -> w333
          frame "Pump" {
            w344 = T10."Enabled" ("Disabled")
            w341 = T10."Disabled and Grayed Out" ("Disabled")
            w343 = enum16{"Auto", "Man", "Error"}."Man" ("Valve 2 Mode")
            n203 = property on="Pump Mode" class="Enum (strict)"("Value"=enum16{"Auto", "Man", "Error"}."Auto" ("Pump Mode")) -> ()  [unwired: 2 in, 2 out]
            n204 = property on="Pump Mode" class="Enum (strict)"("DisabledEnum"=w341) -> ()  [unwired: 2 in, 2 out]
            n205 = property on="Valve 2 Mode" class="Enum (strict)"("DisabledEnum"=w341) -> ()  [unwired: 2 in, 2 out]
            n206 = property on="Valve 1 Mode" class="Enum (strict)"("DisabledEnum"=w341) -> ()  [unwired: 2 in, 2 out]
            n207 = property on="Pump MV" class="Slide (strict)"("DisabledEnum"=w341) -> ()  [unwired: 2 in, 2 out]
            n208 = property on="Valve 1 MV" class="DigNum (strict)"("DisabledEnum"=w344) -> ()  [unwired: 2 in, 2 out]
            n209 = property on="Valve 2 MV" class="DigNum (strict)"("DisabledEnum"=w344) -> ()  [unwired: 2 in, 2 out]
            n210 = property on="Valve 2 Mode" class="Enum (strict)"("Value"=w343) -> ()  [unwired: 2 in, 2 out]
            n211 = property on="Valve 1 Mode" class="Enum (strict)"("Value"=w343) -> ()  [unwired: 2 in, 2 out]
          }
          frame "Valve 1" {
            n212 = property on="Valve 2 MV" class="DigNum (strict)"("DisabledEnum"=T10."Enabled" ("Disabled")) -> ()  [unwired: 2 in, 2 out]
            n213 = property on="Pump Mode" class="Enum (strict)"("DisabledEnum"=T10."Disabled and Grayed Out" ("Disabled")) -> ()  [unwired: 2 in, 2 out]
            n214 = property on="Pump Mode" class="Enum (strict)"("Value"=enum16{"Auto", "Man", "Error"}."Man" ("Pump Mode")) -> ()  [unwired: 2 in, 2 out]
            n215 = property on="Pump MV" class="Slide (strict)"("DisabledEnum"=T10."Enabled" ("Disabled")) -> ()  [unwired: 2 in, 2 out]
            n216 = property on="Valve 1 MV" class="DigNum (strict)"("DisabledEnum"=T10."Disabled and Grayed Out" ("Disabled")) -> ()  [unwired: 2 in, 2 out]
            n217 = property on="Valve 2 Mode" class="Enum (strict)"("DisabledEnum"=T10."Disabled and Grayed Out" ("Disabled")) -> ()  [unwired: 2 in, 2 out]
            n218 = property on="Valve 2 Mode" class="Enum (strict)"("Value"=enum16{"Auto", "Man", "Error"}."Man" ("Valve 2 Mode")) -> ()  [unwired: 2 in, 2 out]
            n219 = property on="Valve 1 Mode" class="Enum (strict)"("DisabledEnum"=T10."Disabled and Grayed Out" ("Disabled")) -> ()  [unwired: 2 in, 2 out]
            n220 = property on="Valve 1 Mode" class="Enum (strict)"("Value"=enum16{"Auto", "Man", "Error"}."Auto" ("Valve 1 Mode")) -> ()  [unwired: 2 in, 2 out]
          }
          frame "Valve 2" {
            n221 = property on="Valve 1 MV" class="DigNum (strict)"("DisabledEnum"=T10."Enabled" ("Disabled")) -> ()  [unwired: 2 in, 2 out]
            n222 = property on="Valve 2 MV" class="DigNum (strict)"("DisabledEnum"=T10."Disabled and Grayed Out" ("Disabled")) -> ()  [unwired: 2 in, 2 out]
            n223 = property on="Pump Mode" class="Enum (strict)"("DisabledEnum"=T10."Disabled and Grayed Out" ("Disabled")) -> ()  [unwired: 2 in, 2 out]
            n224 = property on="Pump Mode" class="Enum (strict)"("Value"=enum16{"Auto", "Man", "Error"}."Man" ("Pump Mode")) -> ()  [unwired: 2 in, 2 out]
            n225 = property on="Pump MV" class="Slide (strict)"("DisabledEnum"=T10."Enabled" ("Disabled")) -> ()  [unwired: 2 in, 2 out]
            n226 = property on="Valve 2 Mode" class="Enum (strict)"("Value"=enum16{"Auto", "Man", "Error"}."Auto" ("Valve 2 Mode")) -> ()  [unwired: 2 in, 2 out]
            n227 = property on="Valve 2 Mode" class="Enum (strict)"("DisabledEnum"=T10."Disabled and Grayed Out" ("Disabled")) -> ()  [unwired: 2 in, 2 out]
            n228 = property on="Valve 1 Mode" class="Enum (strict)"("Value"=enum16{"Auto", "Man", "Error"}."Man" ("Valve 1 Mode")) -> ()  [unwired: 2 in, 2 out]
            n229 = property on="Valve 1 Mode" class="Enum (strict)"("DisabledEnum"=T10."Disabled and Grayed Out" ("Disabled")) -> ()  [unwired: 2 in, 2 out]
          }
          frame "None", Default {
            w366 = T10."Enabled" ("Disabled")
            w369 = T10."Disabled and Grayed Out" ("Disabled")
            w368 = enum16{"Auto", "Man", "Error"}."Man" ("Valve 2 Mode")
            n230 = property on="Pump Mode" class="Enum (strict)"("DisabledEnum"=w369) -> ()  [unwired: 2 in, 2 out]
            n231 = property on="Valve 2 Mode" class="Enum (strict)"("DisabledEnum"=w369) -> ()  [unwired: 2 in, 2 out]
            n232 = property on="Valve 1 Mode" class="Enum (strict)"("DisabledEnum"=w369) -> ()  [unwired: 2 in, 2 out]
            n233 = property on="Valve 1 MV" class="DigNum (strict)"("DisabledEnum"=w366) -> ()  [unwired: 2 in, 2 out]
            n234 = property on="Valve 2 MV" class="DigNum (strict)"("DisabledEnum"=w366) -> ()  [unwired: 2 in, 2 out]
            n235 = property on="Valve 2 Mode" class="Enum (strict)"("Value"=w368) -> ()  [unwired: 2 in, 2 out]
            n236 = property on="Valve 1 Mode" class="Enum (strict)"("Value"=w368) -> ()  [unwired: 2 in, 2 out]
            n237 = property on="Pump Mode" class="Enum (strict)"("Value"=w368) -> ()  [unwired: 2 in, 2 out]
            n238 = property on="Pump MV" class="Slide (strict)"("DisabledEnum"=w366) -> ()  [unwired: 2 in, 2 out]
          }
        }
        n239 = Build Array("OP_OBJECT" ("PV")) -> (w335:string[])
        n240 = call "DataSockets Write.vi"("Data"=w333, "mode"=T7."Write", "Array"=w335, "Main Path"=w337) -> ()  [unwired: 7 in, 1 out]
      }
      frame "SCADA Start" {
        n241 = call "Enqueu Element.vi"("Enum in"=w371, "Message"="Update Display", "Queue in"=w372) -> ()  [unwired: 8 in, 1 out]
        n242 = call "Enqueu Element.vi"("Message"="DataSocket Open", "Queue in"=w374) -> ()  [unwired: 9 in, 1 out]
      }
      frame "Down" {
        n243 = Variant To Data(type=TRUE ("Boolean"), Variant=w375) -> (data=w376:bool)  [unwired: 1 in, 1 out]
        n244 = case shown="True" w376 {
          frame False {
          }
          frame True {
            w385 = "opc://localhost/CoDeSys.OPC.02/PLC1:."  # Main Path
            w384 = T7."Write" ("mode")
            n245 = call "Down.vi"() -> ("Filling time"=w379:dbl)  [unwired: 17 in, 2 out]
            n246 = local read "LLAS On/Off"() -> (w381:bool)
            n247 = Build Array("time_dry_run_interval") -> (w386:string[])
            n248 = Build Array(w379) -> (w378:dbl[])
            n249 = Build Array("DRY_RUN") -> (w382:string[])
            n250 = Build Array(w381) -> (w380:bool[])
            n251 = call "DataSockets Write.vi"("Data"=w378, "mode"=w384, "Array"=w386, "Main Path"=w385) -> ()  [unwired: 7 in, 1 out]
            n252 = call "DataSockets Write.vi"("Data"=w380, "mode"=w384, "Array"=w382, "Main Path"=w385) -> ()  [unwired: 7 in, 1 out]
          }
        }
      }
      frame "Up" {
        n253 = Variant To Data(type=TRUE ("Boolean"), Variant=w388) -> (data=w389:bool)  [unwired: 1 in, 1 out]
        n254 = case shown="True" w389 {
          frame False {
          }
          frame True {
            w394 = "opc://localhost/CoDeSys.OPC.02/PLC1:."  # Main Path
            n255 = call "Up.vi"() -> ("Valve Opening"=w395:dbl, "Pump power"=w399:dbl, "Filling tim"=w398:dbl)  [unwired: 15 in, 2 out]
            n256 = Build Array(w399, w395, w398) -> (w391:dbl[])
            n257 = Build Array("AQ_rOP_engine2" ("PV"), "Open_vlv22" ("PV"), "time_high_lvl_low_tank_interval" ("PV")) -> (w393:string[])
            n258 = call "DataSockets Write.vi"("Data"=w391, "mode"=T7."Write", "Array"=w393, "Main Path"=w394) -> ()  [unwired: 7 in, 1 out]
          }
        }
      }
      frame "PumpDefence" {
        n259 = Variant To Data(type=TRUE ("Boolean"), Variant=w401) -> (data=w402:bool)  [unwired: 1 in, 1 out]
        n260 = case shown="True" w402 {
          frame False {
          }
          frame True {
            w407 = "opc://localhost/CoDeSys.OPC.02/PLC1:."  # Main Path
            n261 = call "PUMP.vi"() -> ("процент открытия выпускного клапна"=w408:dbl, "процент открытия впускного клапна"=w409:dbl)  [unwired: 16 in, 2 out]
            n262 = Build Array(w409, w408) -> (w404:dbl[])
            n263 = Build Array("Open_vlv21", "Open_vlv32") -> (w406:string[])
            n264 = call "DataSockets Write.vi"("Data"=w404, "mode"=T7."Write", "Array"=w406, "Main Path"=w407) -> ()  [unwired: 7 in, 1 out]
          }
        }
      }
      frame "Start Acquisition" {
        n265 = call "Enqueu Element.vi"("Enum in"=w412, "Message"="Update Display", "Queue in"=w414) -> ()  [unwired: 8 in, 1 out]
        n266 = call "Enqueu Element.vi"("Message"=w412, "Queue in"=w415) -> ()  [unwired: 9 in, 1 out]
      }
      frame "Start Identification" {
        n267 = call "Enqueu Element.vi"("Message"=w416, "Queue in"=w417) -> ()  [unwired: 9 in, 1 out]
        n268 = call "Enqueu Element.vi"("Enum in"=w416, "Message"="Update Display", "Queue in"=w418) -> ()  [unwired: 8 in, 1 out]
      }
      frame "Start Autotune" {
        n269 = call "Enqueu Element.vi"("Enum in"=w420, "Message"="Update Display", "Queue in"=w422) -> ()  [unwired: 8 in, 1 out]
        n270 = call "Enqueu Element.vi"("Message"=w420, "Queue in"=w421) -> ()  [unwired: 9 in, 1 out]
      }
      frame "Set PID Coeffs To PLC" {
        n271 = call "Enqueu Element.vi"("Enum in"=w425, "Message"="Update Display", "Queue in"=w426) -> ()  [unwired: 8 in, 1 out]
        n272 = call "Enqueu Element.vi"("Message"=w425, "Queue in"=w424) -> ()  [unwired: 9 in, 1 out]
      }
      frame "Update Display" {
        n273 = Variant To Data(type="", Variant=w430) -> (data=→"State":string)  [unwired: 1 in, 1 out]
      }
      frame "Id method" {
        n274 = Variant To Data(type=enum16{"Transient Response", "Proni"}."Transient Response" ("Select Identification Method"), Variant=w432) -> (data=w433:enum16{"Transient Response", "Proni"})  [unwired: 1 in, 1 out]
        n275 = case shown="\"Proni\"" w433 {
          frame "Transient Response", Default {
            n276 = property on="Prony approximation zone" class="Enum (strict)"("DisabledEnum"=T10."Disabled and Grayed Out" ("Disabled")) -> ()  [unwired: 2 in, 2 out]
          }
          frame "Proni" {
            n277 = property on="Prony approximation zone" class="Enum (strict)"("DisabledEnum"=T10."Enabled" ("Disabled")) -> ()  [unwired: 2 in, 2 out]
          }
        }
      }
      frame "Auto method" {
        n278 = Variant To Data(type=enum32{"Ziegler  -  Nichols", "IMC", "Amigo"}."IMC" ("Select Autotune Method"), Variant=w437) -> (data=w438:enum32{"Ziegler  -  Nichols", "IMC", "Amigo"})  [unwired: 1 in, 1 out]
        n279 = case shown="\"Ziegler  -  Nichols\", Default" w438 {
          frame "Ziegler  -  Nichols", Default {
            n280 = property on="IMC filter value\n(PI > 0,7; PID > 1,7)" class="Slide (strict)"("DisabledEnum"=T10."Disabled and Grayed Out" ("Disabled")) -> ()  [unwired: 2 in, 2 out]
          }
          frame "IMC" {
            n281 = property on="IMC filter value\n(PI > 0,7; PID > 1,7)" class="Slide (strict)"("DisabledEnum"=T10."Enabled" ("Disabled")) -> ()  [unwired: 2 in, 2 out]
          }
          frame "Amigo" {
            n282 = property on="IMC filter value\n(PI > 0,7; PID > 1,7)" class="Slide (strict)"("DisabledEnum"=T10."Disabled and Grayed Out" ("Disabled")) -> ()  [unwired: 2 in, 2 out]
          }
        }
      }
      frame "Exit" {
        w443 = TRUE
        n283 = call "Enqueu Element.vi"("Boolean"=w443, "Message"=w444, "Queue in"=w445) -> ()  [unwired: 8 in, 1 out]
        n284 = call "Enqueu Element.vi"("Boolean"=w443, "Message"="Close DataSockets", "Queue in"=w446) -> ()  [unwired: 8 in, 1 out]
      }
    }
  }
  n285 = while {
    tunnel: w6 -> [w453]
    shift-right: [w451] -> _
    shift-left: _ -> [w450]
    stop <- w448 stop-if-true
    # "Identification And PID Autotune"
    n286 = Dequeue Element(queue=w453) -> (queue out=w449:refnum<queue>, element=w454:T6)  [unwired: 2 in, 2 out]
    n287 = Unbundle By Name(w454) -> ("Message"=w452:string, "Enum"=w447:variant)
    n288 = case shown="\"Start Acquisition\"" w452 {
      tunnel: [dbl[][] [] ("Data Out") w467 _ _ _ _ _] -> w451
      tunnel: w450 -> [_ w466 _ _ _ _ _]
      tunnel: w449 -> [_ w463 w493 w503 _ _ _]
      tunnel: [_ _ _ _ _ _ TRUE] -> w448
      tunnel: w447 -> [_ _ _ _ _ w530 _]
      frame "Wait For Event", Default {
      }
      frame "Start Acquisition" {
        n289 = case shown="\"Valve 1\"" "Manipulated Variable (MV)" {
          tunnel: "Control action level" -> [w471 w475 w479 _]
          frame "Pump", Default {
            n290 = In Range and Coerce(upper limit=1.0, x=w471, lower limit=0.0) -> (coerced(x)=w470:dbl)  [unwired: 1 out]
            n291 = local write "Pump MV"(w470) -> ()
          }
          frame "Valve 1" {
            n292 = In Range and Coerce(upper limit=1.0, x=w475, lower limit=0.0) -> (coerced(x)=w472:dbl)  [unwired: 1 out]
            n293 = local write "Valve 1 MV"(w472) -> ()
          }
          frame "Valve 2" {
            n294 = In Range and Coerce(upper limit=1.0, x=w479, lower limit=0.0) -> (coerced(x)=w476:dbl)  [unwired: 1 out]
            n295 = local write "Valve 2 MV"(w476) -> ()
          }
          frame "None" {
          }
        }
        n296 = case shown="\"Flow 2\"" "Process Variable (PV)" {
          tunnel: [_ w480 w481 w482] -> w457
          frame "None", Default {
          }
          frame "Flow 1" {
            n297 = local read "Flow meter N1"() -> (w480:dbl)
          }
          frame "Flow 2" {
            n298 = local read "Flow meterN2"() -> (w481:dbl)
          }
          frame "Level" {
            n299 = local read "Level N"() -> (w482:dbl)
          }
        }
        n300 = call "Step Responsevi.vi"("Number"="Transient response \nrecord ends in repetitions", "dt, msec"="dt, msec", "PV"=w457, "Data In"=w466) -> ("Complete Data Acquisition"=w462:bool, "Data Out"=w467:dbl[][])  [unwired: 6 in]
        "Transient response database" <- w467
        n301 = feedback #3() -> (w456:dbl[])  [unwired: 1 in]
        n302 = Build Array (concatenate)(w456, w457) -> (w458:dbl[])
        "Waveform Graph" <- w458
        n303 = feedback-in #3(w458) -> ()
        n304 = case shown="True" w462 {
          tunnel: w463 -> [w487 w489]
          frame True {
            w483 = 1.0 ("Valve 1 MV")
            n305 = local write "Pump MV"(0.0 ("Pump MV")) -> ()
            n306 = local write "Valve 1 MV"(w483) -> ()
            n307 = local write "Valve 2 MV"(w483) -> ()
            n308 = call "Enqueu Element.vi"("Enum in"="Acquisition Completed " ("Message"), "Message"="Update Display", "Queue in"=w487) -> ()  [unwired: 8 in, 1 out]
          }
          frame False {
            n309 = call "Enqueu Element.vi"("Message"="Start Acquisition", "Queue in"=w489) -> ()  [unwired: 9 in, 1 out]
          }
        }
      }
      frame "Start Identification" {
        n310 = local read "Control action level"() -> (w490:dbl)
        n311 = local read "Transient response database"() -> (w500:dbl[][])
        n312 = call "Identification.vi"("MVEBRA"=w490, "Data For Ident From OPC"=w500, "Prony\n approximation zone"="Prony approximation zone", "Select Method"="Select Identification Method") -> ("Control object parameters  W(p) out"=w499:T11, "Аverage error"=→"Аverage error":dbl, "Xoutput"=→"Identification X":dbl[], "Array"=→"Initial graph and object identification graph":T12)  [unwired: 8 in]
        n313 = call "Enqueu Element.vi"("Enum in"="Identification Completed" ("Message"), "Message"="Update Display", "Queue in"=w493) -> ()  [unwired: 8 in, 1 out]
        n314 = local write "Identified First - Order process + Deadtime transfer function"(w499) -> ()
      }
      frame "Start Autotune" {
        n315 = Bundle By Name(cluster=cluster{"P1":dbl, "P2":dbl, "P3":dbl} {"P1"=0.0, "P2"=0.0, "P3"=0.0}, "P1"="P1", "P2"="P2", "P3"="P3") -> (w504:cluster{"P1":dbl, "P2":dbl, "P3":dbl})
        n316 = call "Enqueu Element.vi"("Enum in"="Autotune Completed" ("Message"), "Message"="Update Display", "Queue in"=w503) -> ()  [unwired: 8 in, 1 out]
        n317 = call "Autotune.vi"("PID Coeffs"=w504, "Parameters of Filter\n(PI > 0,7; PID > 1,7) in"="IMC filter value\n(PI > 0,7; PID > 1,7)", "Parameters of the control object W(p)"="Identified First - Order process + Deadtime transfer function", "Selecting the type of regulator  \nfor Ziegler–Nichols method"="Type of controller", "Settings Methods Panel"="Select Autotune Method") -> ("P3"=w513:dbl, "P2"=w512:dbl, "P1"=w511:dbl, "Parameters of Filter\n(PI > 0,7; PID > 1,7) out"=w516:dbl)  [unwired: 3 in]
        n318 = local write "P1"(w511) -> ()
        n319 = local write "P2"(w512) -> ()
        n320 = local write "P3"(w513) -> ()
        n321 = local write "IMC filter value\n(PI > 0,7; PID > 1,7)"(w516) -> ()
      }
      frame "Set PID Coeffs To PLC" {
        w524 = "opc://localhost/CoDeSys.OPC.02/PLC1:."  # Main Path
        n322 = local read "P1"() -> (w521:dbl)
        n323 = local read "P2"() -> (w520:dbl)
        n324 = local read "P3"() -> (w519:dbl)
        n325 = Build Array(w521, w520, w519) -> (w517:dbl[])
        n326 = call "DataSockets Open.vi"("mode"=T7."Write", "Variables"=string[] ["rKp", "rKi", "rKd"], "Main Path"=w524) -> ("Array"=w518:refnum<k13>[])  [unwired: 7 in, 1 out]
        n327 = for {
          tunnel: w517 -> [w529] mode=indexing
          tunnel: w518 -> [w528] mode=indexing
          tunnel: [w525] -> _ mode=indexing
          n328 = DataSocket Write(10:w529, 11:w528) -> (0:w526:errorcluster, 3:w527:refnum<k13>)  [unwired: 2 in, 1 out]
          n329 = DataSocket Close(8:w526, 11:w527) -> (0:w525:errorcluster)  [unwired: 1 in, 1 out]
        }
      }
      frame "Update Display" {
        n330 = Variant To Data(type="" ("data"), Variant=w530) -> (data=w532:string)  [unwired: 1 in, 1 out]
        n331 = local write "State"(w532) -> ()
      }
      frame "Exit" {
      }
    }
  }
